vi "FS Body Cuboid.vi"(8 "Body #":i32=1, 9 "Cuboid":T1={"Point 1"={"x"=0.0, "y"=0.0, "z"=0.0}, "Point 2"={"x"=1.0, "y"=1.0, "z"=1.0}}, 11 "Feature In":string="FeatureScript 1247;\nimport(path : \"onshape/std/geometry.fs\", version : \"1247.0\");\n\nannotation { \"Feature Type Name\" : \"LabVIEW Feature\" }\nexport const myFeature = defineFeature(function(context is Context, id is Id, definition is map)\n    precondition\n    {\n        // Define the parameters of the feature type\n    }\n    {\n        // Define the function's action\n\nvar sketch1 = newSketch(context, id + \"sketch1\", {\n                \"sketchPlane\" : qCreatedBy(makeId(\"Top\"), EntityType.FACE)\n        });\n        // Create sketch entities here\n        skRectangle(sketch1, \"rectangle1\", {\n                \"firstCorner\" : vector(0, 0) * inch,\n                \"secondCorner\" : vector(3, 4) * inch\n        });\n        \n        skSolve(sketch1);\n    });") -> (3 "Feature Out":string="FeatureScript 1247;\nimport(path : \"onshape/std/geometry.fs\", version : \"1247.0\");\n\nannotation { \"Feature Type Name\" : \"LVFeat1\" }\nexport const myFeature = defineFeature(function(context is Context, id is Id, definition is map)\n    precondition\n    {\n        // Define the parameters of the feature type\n    }\n    {\n        // Define the function's action\n       fEllipsoid(context, id + \"ellipsoid1\", {\n                \"center\" : vector(5, 0, 0) * inch,\n                \"radius\" : vector(3, 3, 3) * inch,\n        });\n\nvar sketch1 = newSketch(context, id + \"sketch1\", {\n                \"sketchPlane\" : qCreatedBy(makeId(\"Top\"), EntityType.FACE)\n        });\n        // Create sketch entities here\n        skRectangle(sketch1, \"rectangle1\", {\n                \"firstCorner\" : vector(0, 0) * inch,\n                \"secondCorner\" : vector(3, 4) * inch\n        });\n        \n        skSolve(sketch1);\n    });")   [LabVIEW 2019]
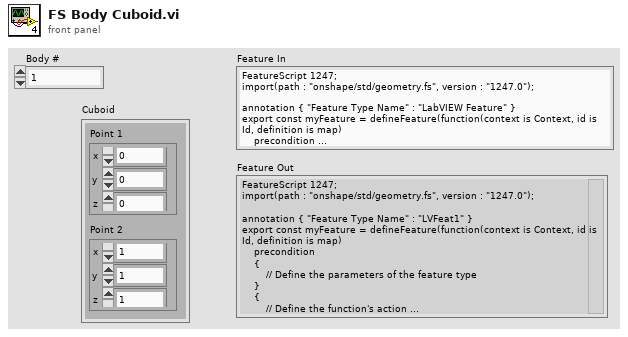
[diagram p1: front panel]
types:
  T1 = cluster{"Point 1":cluster{"x":dbl, "y":dbl, "z":dbl}, "Point 2":cluster{"x":dbl, "y":dbl, "z":dbl}}
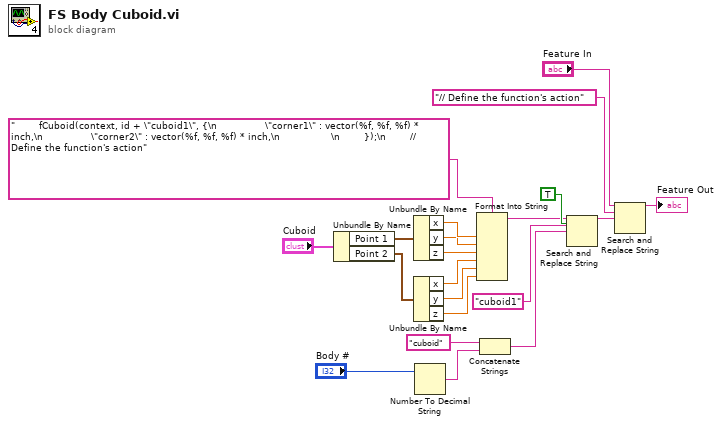
[diagram p0: block diagram]
diagram:
  n1 = Unbundle By Name("Cuboid") -> ("Point 1"=w16:cluster{"x":dbl, "y":dbl, "z":dbl}, "Point 2"=w15:cluster{"x":dbl, "y":dbl, "z":dbl})
  n2 = Unbundle By Name(w16) -> ("x"=w8:dbl, "y"=w7:dbl, "z"=w6:dbl)
  n3 = Unbundle By Name(w15) -> ("x"=w5:dbl, "y"=w4:dbl, "z"=w3:dbl)
  n4 = Number To Decimal String(number="Body #") -> (decimal integer string=w10:string)  [unwired: 1 in]
  n5 = Format Into String(format string="        fCuboid(context, id + \"cuboid1\", {\n                \"corner1\" : vector(%f, %f, %f) * inch,\n                \"corner2\" : vector(%f, %f, %f) * inch,\n                 \n        });\n        // Define the function's action" ("search string"), w8, w7, w6, w5, w4, w3) -> (resulting string=w2:string)  [unwired: 2 in, 1 out]
  n6 = Concatenate Strings("cuboid" ("regular expression"), w10) -> (w11:string)
  n7 = Search and Replace String(replace all?=TRUE ("replace all? (F)"), input string=w2, search string="cuboid1" ("regular expression"), replace string=w11) -> (result string=w9:string)  [unwired: 4 in, 3 out]
  n8 = Search and Replace String(input string="Feature In", search string="// Define the function's action", replace string=w9) -> (result string=→"Feature Out":string)  [unwired: 5 in, 3 out]
